vi "Resize_img.vi"(0 "w2":i32, 1 "w1":i32, 3 "h2":i32, 4 "h1":i32, 5 "img_in":i32[][](array[numeric])) -> (2 "img_out":i32[][](array[numeric]))   [LabVIEW 2016]
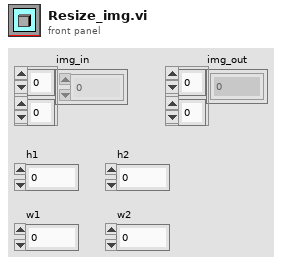
[diagram p1: front panel]
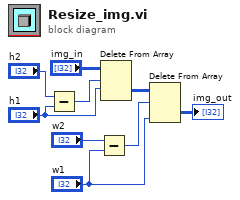
[diagram p0: block diagram]
diagram:
  n1 = Subtract(x="h2", y="h1") -> (x-y=w6:i32)
  n2 = Subtract(x="w2", y="w1") -> (x-y=w3:i32)
  n3 = Delete From Array(array="img_in", length=w6, index (row)="h1") -> (deleted portion=w5:i32[][])  [unwired: 1 in, 1 out]
  n4 = Delete From Array(array=w5, length=w3, index (col)="w1") -> (deleted portion=→"img_out":i32[][])  [unwired: 1 in, 1 out]
